vi "process.vi"(8 "error in (no error)":errorcluster, 10 "Sync":refnum<notifier>, 11 "Session in":refnum<class "Session.lvclass">) -> (0 "error out":errorcluster, 3 "Session out":refnum<class "Session.lvclass">)   [LabVIEW 2013, in "MQTT Base.lvlib" / "Session.lvclass"]
uses:
  Session.lvclass
  Session.lvclass/Session.ctl
  Session Disconnection Reason -- enum.ctl
  <vilib>/LabVIEW Open Source Project/MQTT Control Packets/Control Packets/ControlPacket/ControlPacket.lvclass
  <vilib>/LabVIEW Open Source Project/MQTT Control Packets/Control Packets/MQTT_311/MQTTVersion.lvclass
  MQTT_Connection/Connection/Connection.lvclass
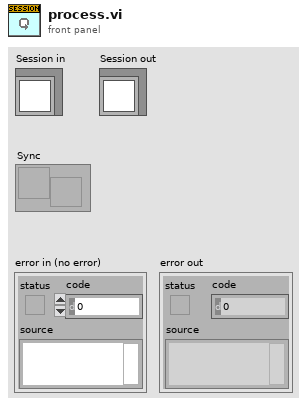
[diagram p1: front panel]
types:
  T1 = typedef "MQTT Base.lvlib/Session.lvclass/Session Disconnection Reason -- enum.ctl" = enum16{"Normal Stop", "Protocol Violation", "Disconnected by Peer"}
  T2 = typedef "MQTT Base.lvlib/MQTT_Base.lvclass/Response -- cluster.ctl" = cluster{"Packet":refnum<class "ControlPacket.lvclass">, "Protocol Error":errorcluster, "disconnect session":bool, "[ACK]":refnum<notifier>[]}
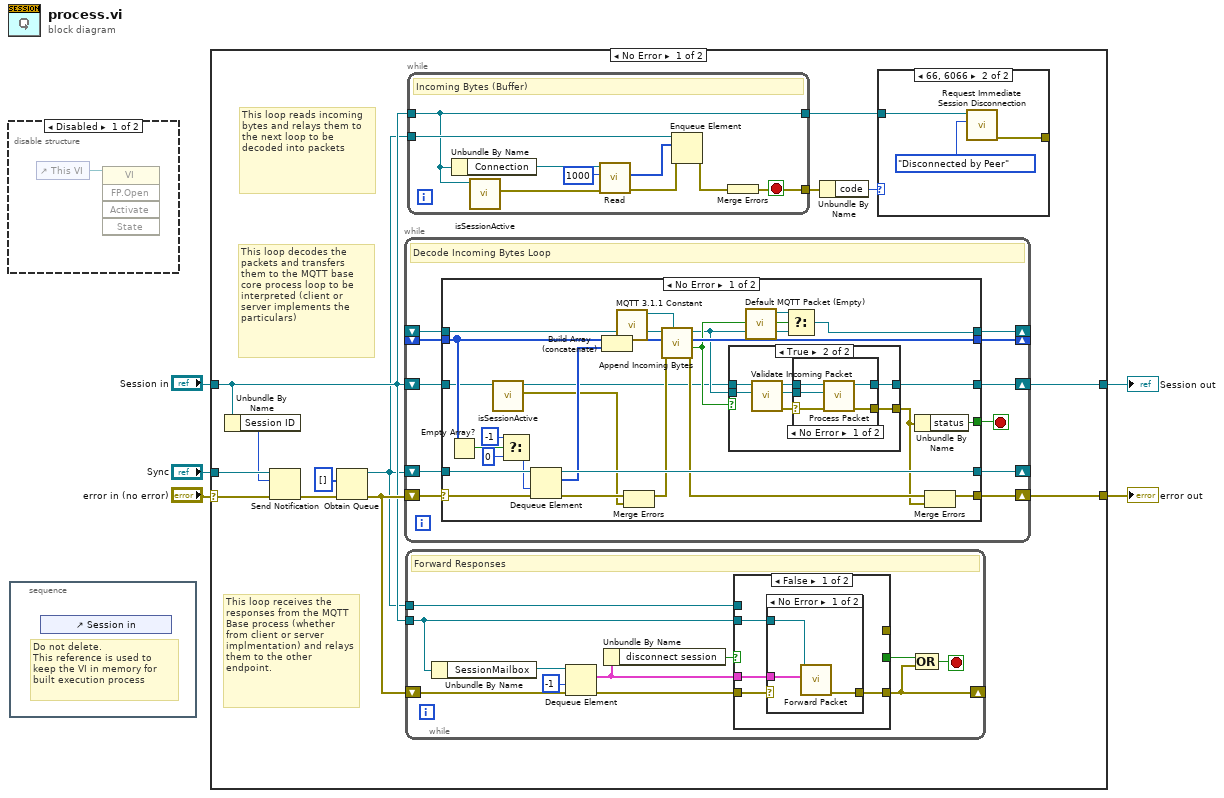
[diagram p0: block diagram]
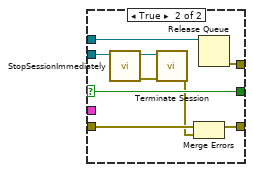
[diagram p4: hidden frame]
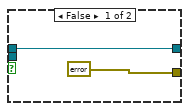
[diagram p6: hidden frame]
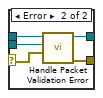
[diagram p7: hidden frame]
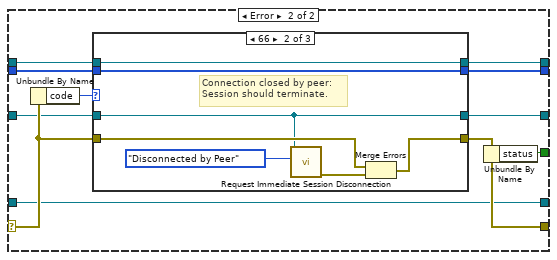
[diagram p8: hidden frame]
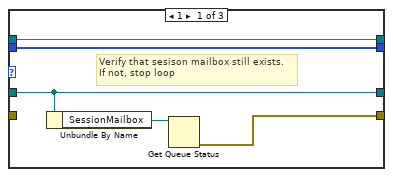
[diagram p9: hidden frame]
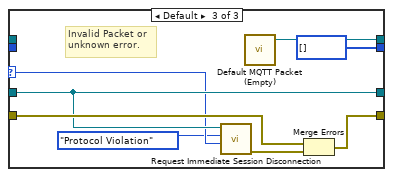
[diagram p10: hidden frame]
diagram:
  n1 = disable-structure shown="Disabled" {
    frame Disabled {
      n2 = control-ref of="This VI"() -> (w6:refnum<vi>)
      n3 = invoke class="VI" method="FP.Open"(reference=w6) -> ()  [unwired: 4 in, 5 out]
    }
    frame Enabled {
    }
  }
  n4 = stacked-sequence {
    frame #0 {
      # "Do not delete.\nThis reference is used to keep the VI in memory for built execution process"
      n5 = control-ref of="Session in"() -> ()  [unwired: 1 out]
    }
  }
  n6 = case shown="No Error" "error in (no error)" {
    selector: "error in (no error)" -> [w18 w149]
    tunnel: [w11 w149] -> w1
    tunnel: [w13 w148] -> w3
    tunnel: "Session in" -> [w9 w148]
    tunnel: "Sync" -> [w19 _]
    frame No Error {
      # "This loop receives the responses from the MQTT Base process (whether from client or server implmentation) and relays them to the other endpoint."
      # "This loop decodes the packets and transfers them to the MQTT base core process loop to be interpreted (client or server implements the particulars)"
      # "This loop reads incoming bytes and relays them to the next loop to be decoded into packets"
      n7 = Unbundle By Name(w9) -> ("Session ID"=w10:i32)
      n8 = Send Notification(notification=w10, notifier=w19, error in (no error)=w18) -> (error out=w12:errorcluster)  [unwired: 1 out]
      n9 = Obtain Queue(element data type=u8[] [] ("Remaining Packets"), error in (no error)=w12) -> (queue out=w7:refnum<queue>, error out=w17:errorcluster)  [unwired: 3 in, 1 out]
      n10 = while {
        shift-right: [w68] -> _
        shift-left: _ -> [w67]
        shift-right: [w66] -> w11
        shift-left: w17 -> [w65]
        shift-right: [w69] -> _
        shift-left: _ -> [w70]
        shift-right: [w62] -> _
        shift-left: w7 -> [w63]
        shift-right: [w60] -> w13
        shift-left: w9 -> [w61]
        stop <- w64 stop-if-true
        # "Decode Incoming Bytes Loop"
        n11 = case shown="No Error" w65 {
          selector: w65 -> [w90 w125]
          tunnel: w70 -> [w97 w123]
          tunnel: [w82 w127] -> w69
          tunnel: [w95 w126] -> w68
          tunnel: w67 -> [w87 w117]
          tunnel: [w88 w122] -> w66
          tunnel: [w76 w121] -> w64
          tunnel: w63 -> [w94 w120]
          tunnel: [w93 w120] -> w62
          tunnel: w61 -> [w73 w119]
          tunnel: [w78 w118] -> w60
          frame No Error {
            # "No Error"
            n12 = Empty Array?(array=w87) -> (empty?=w86:bool)
            n13 = call "isSessionActive.vi"("Session in"=w73) -> ("error out"=w71:errorcluster, "Session out"=w72:refnum<class "Session.lvclass">)  [unwired: 9 in]
            n14 = Select(t=-1 ("timeout in ms (-1)"), s=w86, f=0) -> (s? t:f=w84:i32)
            n15 = Dequeue Element(queue=w94, timeout in ms (-1)=w84, error in (no error)=w90) -> (queue out=w93:refnum<queue>, element=w92:u8[], error out=w75:errorcluster)  [unwired: 1 out]
            n16 = Build Array (concatenate)(w87, w92) -> (w91:u8[])
            n17 = call <vilib>:"MQTT 3.1.1 Constant.vi"() -> ("MQTT 3.1.1"=w96:refnum<class "MQTTVersion.lvclass">)  [unwired: 11 in]
            n18 = Merge Errors(w75, w71) -> (w74:errorcluster)
            n19 = call <vilib>:"Append Incoming Bytes.vi"("MQTT Version (3.1.1)"=w96, "error in (no error)"=w74, "Incoming Packets"=w91, "Incomplete ControlPacket"=w97) -> ("error out"=w89:errorcluster, "Complete Packet"=w80:bool, "Remaining Packets"=w95:u8[], "ControlPacket"=w79:refnum<class "ControlPacket.lvclass">)  [unwired: 4 in]
            n20 = case shown="True" w80 {
              tunnel: [errorcluster {"status"=FALSE, "code"=0, "source"=""} ("error out") w100] -> w77
              tunnel: w79 -> [_ w106]
              tunnel: w72 -> [w98 w105]
              tunnel: [w98 w101] -> w78
              frame False {
                # "No Packet received"
              }
              frame True {
                # "Packet Received"
                n21 = call-dynamic "Validate Incoming Packet.vi"("ControlPacket"=w106, "Session in"=w105) -> ("error out"=w102:errorcluster, "ControlPacket out"=w103:refnum<class "ControlPacket.lvclass">, "Session out"=w104:refnum<class "Session.lvclass">)  [unwired: 7 in]
                n22 = case shown="No Error" w102 {
                  selector: w102 -> [w107 w114]
                  tunnel: [w108 w112] -> w101
                  tunnel: w104 -> [w111 w116]
                  tunnel: w103 -> [w110 w115]
                  tunnel: [w109 w113] -> w100
                  frame No Error {
                    n23 = call-dynamic "Process Packet.vi"("error in (no error)"=w107, "Incoming Packet"=w110, "Session in"=w111) -> ("error out"=w109:errorcluster, "Session out"=w108:refnum<class "Session.lvclass">)  [unwired: 7 in]
                  }
                  frame Error {
                    n24 = call "Handle Packet Validation Error.vi"("Packet Validation Error"=w114, "ControlPacket"=w115, "Session in"=w116) -> ("error out"=w113:errorcluster, "Session out"=w112:refnum<class "Session.lvclass">)  [unwired: 7 in]
                  }
                }
              }
            }
            n25 = call <vilib>:"Default MQTT Packet (Empty).vi"() -> ("No Packet"=w81:refnum<class "ControlPacket.lvclass">)  [unwired: 11 in]
            n26 = Select(t=w81, s=w80, f=w79) -> (s? t:f=w82:refnum<class "ControlPacket.lvclass">)
            n27 = Unbundle By Name(w77) -> ("status"=w76:bool)
            n28 = Merge Errors(w89, w77) -> (w88:errorcluster)
          }
          frame Error {
            # "Handle Error"
            n29 = Unbundle By Name(w125) -> ("code"=w124:i32)
            n30 = case shown="66" w124 {
              selector: w124 -> [_ _ w142]
              tunnel: [w131 w139 w145] -> w127
              tunnel: w125 -> [_ w137 w147]
              tunnel: [w128 w136 w146] -> w122
              tunnel: [w130 w138 u8[] [] ("Remaining Packets")] -> w126
              tunnel: w123 -> [w131 w139 _]
              tunnel: w119 -> [w129 w134 w143]
              tunnel: [w129 w134 w143] -> w118
              tunnel: w117 -> [w130 w138 _]
              frame 1 {
                # "Verify that sesison mailbox still exists.\nIf not, stop loop"
                n31 = Unbundle By Name(w129) -> ("SessionMailbox"=w132:refnum<queue>)
                n32 = Get Queue Status(queue=w132) -> (error out=w128:errorcluster)  [unwired: 2 in, 7 out]
              }
              frame 66 {
                # "Connection closed by peer:\nSession should terminate."
                n33 = call "Request Immediate Session Disconnection.vi"("Disconnection Reason"=Session_Disconnection_Reason_--_enum."Disconnected by Peer", "Session in"=w134) -> ("error out"=w135:errorcluster)  [unwired: 8 in, 1 out]
                n34 = Merge Errors(w137, w135) -> (w136:errorcluster)
              }
              frame Default {
                # "Invalid Packet or\nunknown error."
                n35 = call "Request Immediate Session Disconnection.vi"("Protocol Violation Error Code"=w142, "Disconnection Reason"=Session_Disconnection_Reason_--_enum."Protocol Violation", "Session in"=w143) -> ("error out"=w141:errorcluster)  [unwired: 7 in, 1 out]
                n36 = call <vilib>:"Default MQTT Packet (Empty).vi"() -> ("No Packet"=w145:refnum<class "ControlPacket.lvclass">)  [unwired: 11 in]
                n37 = Merge Errors(w147, w141) -> (w146:errorcluster)
              }
            }
            n38 = Unbundle By Name(w122) -> ("status"=w121:bool)
          }
        }
      }
      n39 = while {
        tunnel: w9 -> [w26]
        shift-right: [w23] -> _
        shift-left: w17 -> [w27]
        tunnel: w7 -> [w20]
        stop <- w22 stop-if-true
        # "Forward Responses"
        n40 = Unbundle By Name(w26) -> ("SessionMailbox"=w30:refnum<queue>)
        n41 = Dequeue Element(queue=w30, timeout in ms (-1)=-1, error in (no error)=w27) -> (element=w25:T2, error out=w28:errorcluster)  [unwired: 2 out]
        n42 = Unbundle By Name(w25) -> ("disconnect session"=w24:bool)
        n43 = case shown="False" w24 {
          selector: w24 -> [_ w47]
          tunnel: w28 -> [w34 w45]
          tunnel: [w33 w44] -> w23
          tunnel: w26 -> [w32 w46]
          tunnel: w25 -> [w31 _]
          tunnel: [_ w47] -> w21
          tunnel: w20 -> [_ w40]
          tunnel: [_ w39] -> _
          frame False {
            n44 = case shown="No Error" w34 {
              selector: w34 -> [_ w38]
              tunnel: w31 -> [w36 _]
              tunnel: [w35 w38] -> w33
              tunnel: w32 -> [w37 _]
              frame No Error {
                n45 = call-dynamic "Forward Packet.vi"("Response"=w36, "Session in"=w37) -> ("error out"=w35:errorcluster)  [unwired: 9 in]
              }
              frame Error {
              }
            }
          }
          frame True {
            n46 = call "StopSessionImmediately.vi"("Session in"=w46) -> ("error out"=w42:errorcluster, "Session out"=w43:refnum<class "Session.lvclass">)  [unwired: 9 in]
            n47 = call "Terminate Session.vi"("error in (no error)"=w42, "Session in"=w43) -> ("error out"=w41:errorcluster)  [unwired: 7 in, 2 out]
            n48 = Merge Errors(w45, w41) -> (w44:errorcluster)
            n49 = Release Queue(queue=w40) -> (error out=w39:errorcluster)  [unwired: 2 in, 2 out]
          }
        }
        n50 = Compound Arithmetic op=OR(w21, w23) -> (w22:bool)
      }
      n51 = while {
        tunnel: w9 -> [w51]
        tunnel: [w57] -> w15
        tunnel: [w51] -> w8
        tunnel: w7 -> [w59]
        stop <- w57 stop-if-true
        # "Incoming Bytes (Buffer)"
        n52 = Unbundle By Name(w51) -> ("Connection"=w56:refnum<class "Connection.lvclass">)
        n53 = call "isSessionActive.vi"("Session in"=w51) -> ("error out"=w52:errorcluster)  [unwired: 9 in, 1 out]
        n54 = call "Read.vi"("error in (no error)"=w52, "bytes to read (100)"=1000, "TCPConnection in"=w56) -> ("error out"=w53:errorcluster, "Bytes"=w55:u8[])  [unwired: 4 in, 3 out]
        n55 = Enqueue Element(queue=w59, element=w55, error in (no error)=w53) -> (error out=w58:errorcluster)  [unwired: 1 in, 2 out]
        n56 = Merge Errors(w58) -> (w57:errorcluster)
      }
      n57 = Unbundle By Name(w15) -> ("code"=w16:i32)
      n58 = case shown="66, 6066" w16 {
        tunnel: w8 -> [_ w50]
        tunnel: [_ w48] -> _
        frame Default {
        }
        frame 66, 6066 {
          n59 = call "Request Immediate Session Disconnection.vi"("Disconnection Reason"=Session_Disconnection_Reason_--_enum."Disconnected by Peer", "Session in"=w50) -> ("error out"=w48:errorcluster)  [unwired: 8 in, 1 out]
        }
      }
    }
    frame Error {
    }
  }
  "error out" <- w1
  "Session out" <- w3
